vi "Write port.vi"(5 "port":u16=9090, 9 "Downloader in":refnum<class "Downloader.lvclass">) -> (3 "Downloader out":refnum<class "Downloader.lvclass">)   [LabVIEW 2014, in "Downloader.lvclass"]
uses:
  Downloader.lvclass
  Downloader.lvclass/Downloader.ctl
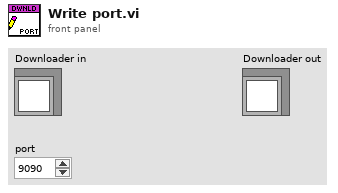
[diagram p1: front panel]
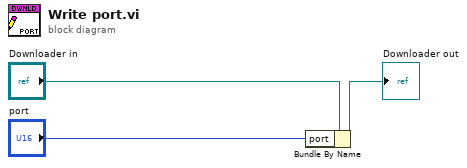
[diagram p0: block diagram]
diagram:
  n1 = Bundle By Name(cluster="Downloader in", "port"="port") -> (→"Downloader out":refnum<class "Downloader.lvclass">)
